vi "zadanie_3.vi"() -> ()   [LabVIEW 2023]
panel:
  in  "stop":bool
  in  "OK Button":bool
  in  "Boolean":bool
  out "Tank":dbl(slide) scale=0.0..1000.0
  # "Napelniaj"
  # "ON"
  # "OFF"
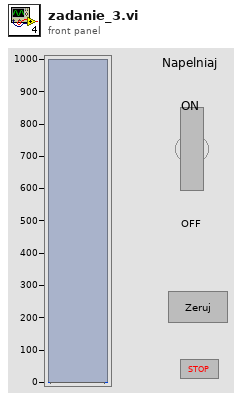
[diagram p1: front panel]
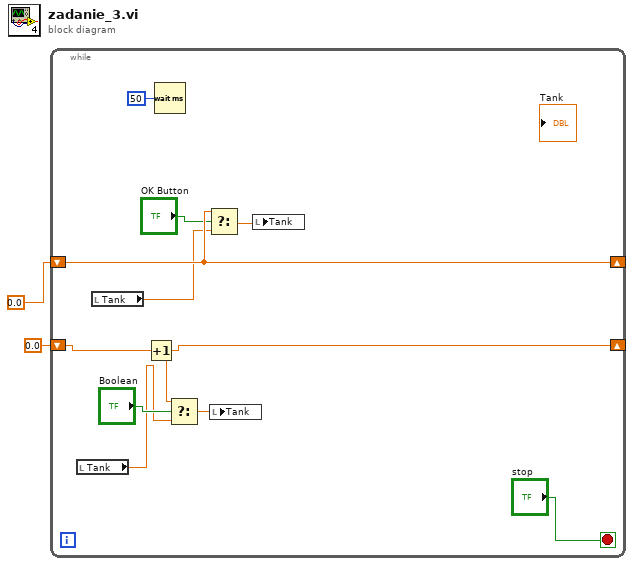
[diagram p0: block diagram]
diagram:
  n1 = while {
    shift-right: [w11] -> _
    shift-left: 0.0 -> [w11]
    shift-right: [w7] -> _
    shift-left: 0.0 -> [w8]
    stop <- "stop" stop-if-true
    n2 = local read "Tank"() -> (w3:dbl)
    n3 = local read "Tank"() -> (w6:dbl)
    n4 = Increment(x=w8) -> (x+1=w7:dbl)
    n5 = Wait (ms)(milliseconds to wait=u32 50) -> ()  [unwired: 1 out]
    n6 = Select(t=w7, s="Boolean", f=w3) -> (s? t:f=w4:dbl)
    n7 = Select(t=w11, s="OK Button", f=w6) -> (s? t:f=w5:dbl)
    n8 = local write "Tank"(w4) -> ()
    n9 = local write "Tank"(w5) -> ()
  }
